vi "Get Default Config Path.vi"(8 "error in (no error)":errorcluster) -> (0 "error out":errorcluster, 3 "appended path":path)   [LabVIEW 2020, in "Process.lvclass"]
doc: "Generates the default configuration path. \nWhen called from the development environement, the default config path is the /Config relative to the project path.\nWhen called from a built exe the default config path is at C:\\Users\\<username>\\AppData\\Local\\<CompanyName>\\<ProductName> where company name and product name are the ones configured in the build specification.\nOn Linux the default config directory is \\home\\lvuser\\natinst\\bin\\config."
uses:
  Process.lvclass
  <vilib>/Utility/sysdir.llb/System Directory Type.ctl
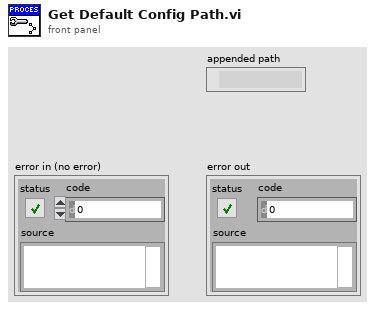
[diagram p1: front panel]
types:
  T1 = typedef "System Directory Type.ctl" = i32
  T2 = typedef "FileVersionInformation.ctl" = cluster{"FileVersion":string, "ProductName":string, "InternalName":string, "CompanyName":string, "LegalCopyright":string, "FileDescription":string}
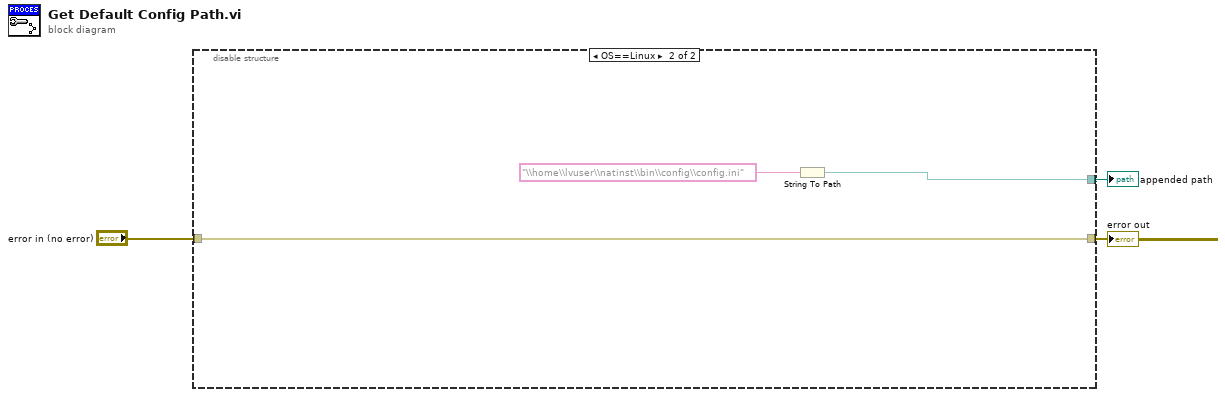
[diagram p0: block diagram]
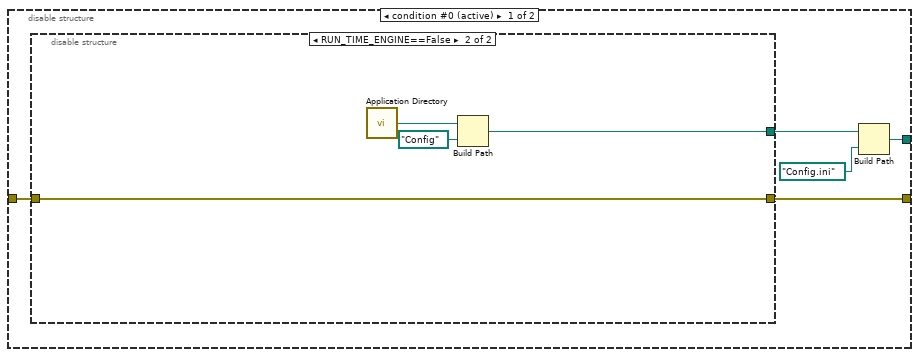
[diagram p2: hidden frame]
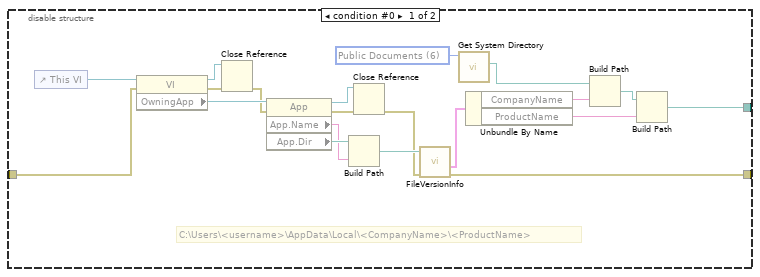
[diagram p3: hidden frame]
diagram:
  n1 = disable-structure shown="OS==Linux" {
    disable-tunnel: "error in (no error)" -> [w8 w35]
    disable-tunnel: [w7 w35] -> w3
    disable-tunnel: [w5 w34] -> w1
    frame condition #0 (active) {
      n2 = disable-structure shown="RUN_TIME_ENGINE==False" {
        disable-tunnel: w8 -> [w18 w29]
        disable-tunnel: [w17 w29] -> w7
        disable-tunnel: [w9 w30] -> w6
        frame condition #0 {
          w16 = T1 6 items=["User Home"=0, "User Desktop"=1, "User Documents"=2, "User Application Data"=3, "User Preferences"=4, "User Temporary"=5, "Public Documents"=6, "Public Application Data"=7, "Public Preferences"=8, "Public Cache"=13, "System Core Libraries"=9, "System Installed Libraries"=10, "Application Files"=11, "Boot Volume Root"=12] ("system directory type")
          # "C:\\Users\\<username>\\AppData\\Local\\<CompanyName>\\<ProductName>"
          n3 = control-ref of="This VI"() -> (w10:refnum<vi>)
          n4 = property class="VI"(reference=w10, error in=w18) -> (reference out=w21:refnum<vi>, error out=w23:errorcluster, "OwningApp"=w28:refnum<vi>)
          n5 = Close Reference(reference=w21, error in (no error)=w23) -> (error out=w22:errorcluster)
          n6 = property class="App"(reference=w28, error in=w22) -> (reference out=w19:refnum<vi>, error out=w24:errorcluster, "App.Name"=w26:string, "App.Dir"=w27:path)
          n7 = Build Path(base path=w27, name or relative path=w26) -> (appended path=w25:path)
          n8 = Close Reference(reference=w19, error in (no error)=w24) -> (error out=w20:errorcluster)
          n9 = call <vilib>:"FileVersionInfo.vi"("error in (no error)"=w20, "Application Path in"=w25) -> ("error out"=w17:errorcluster, "FileVersionInfo Out"=w15:T2)  [unwired: 6 in, 2 out]
          n10 = call <vilib>:"Get System Directory.vi"("system directory type"=w16) -> ("system directory"=w11:path)  [unwired: 10 in]
          n11 = Unbundle By Name(w15) -> ("CompanyName"=w12:string, "ProductName"=w14:string)
          n12 = Build Path(base path=w11, name or relative path=w12) -> (appended path=w13:path)
          n13 = Build Path(base path=w13, name or relative path=w14) -> (appended path=w9:path)
        }
        frame condition #1 (active) {
          n14 = call <vilib>:"Application Directory.vi"() -> ("Application Directory"=w32:path)
          n15 = Build Path(base path=w32, name or relative path=path "Config") -> (appended path=w30:path)
        }
      }
      n16 = Build Path(base path=w6, name or relative path=path "Config.ini") -> (appended path=w5:path)
    }
    frame condition #1 {
      n17 = String To Path(string="\\home\\lvuser\\natinst\\bin\\config\\config.ini") -> (path=w34:path)
    }
  }
  "appended path" <- w1
  "error out" <- w3
